vi "Read.vi"(8 "error in (no error)":errorcluster, 11 "Boolean Constant in":refnum<class "Boolean.lvclass">) -> (0 "error out":errorcluster, 2 "Boolean":bool, 3 "Boolean Constant out":refnum<class "Boolean.lvclass">)   [LabVIEW 2021, in "Variable.lvlib" / "Boolean.lvclass"]
uses:
  Boolean.lvclass
  Boolean.lvclass/Boolean.ctl
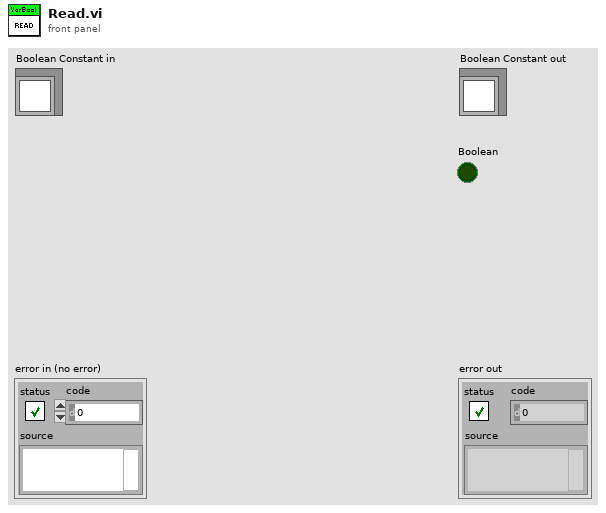
[diagram p1: front panel]
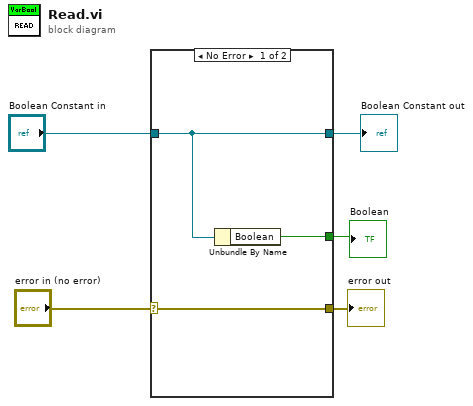
[diagram p0: block diagram]
diagram:
  n1 = case shown="No Error" "error in (no error)" {
    selector: "error in (no error)" -> [w6 w9]
    tunnel: "Boolean Constant in" -> [w7 w10]
    tunnel: [w8 _] -> w4
    tunnel: [w7 w10] -> w3
    tunnel: [w6 w9] -> w1
    frame No Error {
      n2 = Unbundle By Name(w7) -> ("Boolean"=w8:bool)
    }
    frame Error {
    }
  }
  "error out" <- w1
  "Boolean Constant out" <- w3
  "Boolean" <- w4
